vi "Put in mailbox.vi"(6 "Priority? (F)":bool, 8 "error in (no error)":errorcluster, 9 "timeout (100ms)":i32=100, 10 "Message":variant, 11 "Queue in":refnum<queue>) -> (0 "error out":errorcluster, 1 "timed out?":bool, 3 "Queue out":refnum<queue>)   [LabVIEW 2022 SP3]
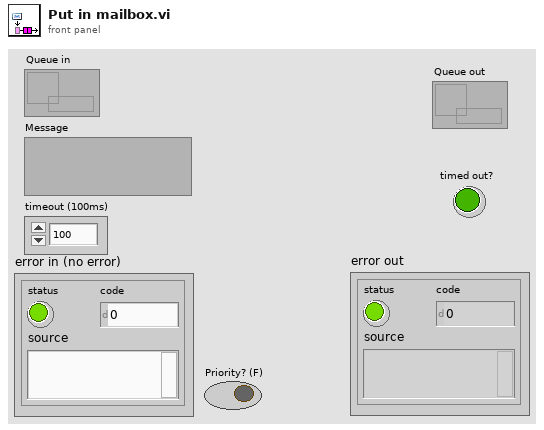
[diagram p1: front panel]
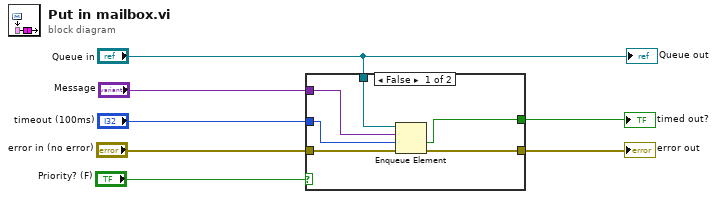
[diagram p0: block diagram]
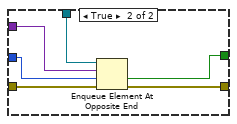
[diagram p2: hidden frame]
diagram:
  n1 = case shown="False" "Priority? (F)" {
    tunnel: "Message" -> [w13 w19]
    tunnel: "error in (no error)" -> [w12 w18]
    tunnel: [w11 w17] -> w3
    tunnel: "timeout (100ms)" -> [w10 w16]
    tunnel: [w9 w15] -> w5
    tunnel: "Queue in" -> [w8 w14]
    frame False {
      n2 = Enqueue Element(queue=w8, element=w13, timeout in ms (-1)=w10, error in (no error)=w12) -> (timed out?=w9:bool, error out=w11:errorcluster)  [unwired: 1 out]
    }
    frame True {
      n3 = Enqueue Element At Opposite End(queue=w14, element=w19, timeout in ms (-1)=w16, error in (no error)=w18) -> (timed out?=w15:bool, error out=w17:errorcluster)  [unwired: 1 out]
    }
  }
  "error out" <- w3
  "timed out?" <- w5
  "Queue out" <- "Queue in"
